vi "Format dotNet response.vi"(7 ".NET Refnum in":refnum<k24>, 11 "error in (no error)":errorcluster) -> (3 "error IO":errorcluster)   [LabVIEW 2015]
uses:
  C:/GitRepo/PerkinElmer/QRD-FW-Server/Sniffer.900/External Dependencies/PerkinElmer.SimplicityServer.LVWrapper.dll
  External Dependencies/PerkinElmer.SimplicityServer.LVWrapper.dll
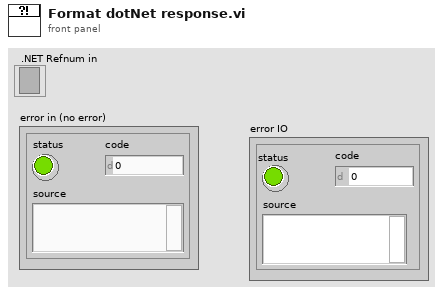
[diagram p1: front panel]
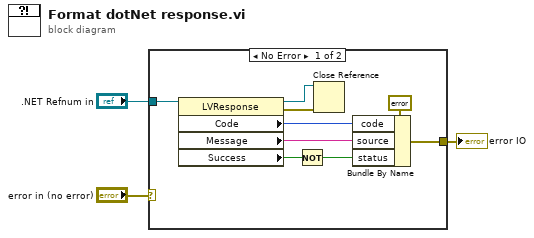
[diagram p0: block diagram]
diagram:
  n1 = case shown="No Error" "error in (no error)" {
    selector: "error in (no error)" -> [_ w13]
    tunnel: ".NET Refnum in" -> [w12 _]
    tunnel: [w7 w13] -> w1
    frame No Error {
      n2 = property class="LVResponse"(reference=w12) -> (reference out=w5:refnum<k24>, error out=w6:errorcluster, "Code"=w10:i32, "Message"=w9:string, "Success"=w8:bool)  [unwired: 1 in]
      n3 = Not(x=w8) -> (.not. x?=w4:bool)
      n4 = Close Reference(reference=w5, error in (no error)=w6) -> ()  [unwired: 1 out]
      n5 = Bundle By Name(cluster=errorcluster {"status"=FALSE, "code"=0, "source"=""} ("error in (no error)"), "code"=w10, "source"=w9, "status"=w4) -> (w7:errorcluster)
    }
    frame Error {
    }
  }
  "error IO" <- w1
